vi "clien fix fix.vi"() -> ()   [LabVIEW 2017]
uses:
  <vilib>/Analysis/Matrix/Datatypes/RealMatrix.ctl
  <vilib>/Platform/TimedLoop/XDataNode/timing_clust.ctl
  <vilib>/Platform/TimedLoop/XDataNode/nitl_modes.ctl
  <vilib>/Platform/TimedLoop/XDataNode/wakeup.ctl
  <vilib>/Analysis/Matrix/Numeric/Multiply/Multiply - RM,RM.vi
  <vilib>/platform/TimedLoop/XDataNode/XDataNode.xnode
  <vilib>/Analysis/Matrix/NI_Matrix.lvlib
  <vilib>/Platform/TimedLoop/XDataNode/XDNodeRunTimeDep.lvlib
panel:
  out "appended array":T1
  in  "Array 8":dbl[](array[numeric])
  in  "Array 7":dbl[](array[numeric])
  in  "Array 6":dbl[](array[numeric])
  in  "Array 5":dbl[](array[numeric])
  in  "Array 4":dbl[](array[numeric])
  in  "Array 3":dbl[](array[numeric])
  in  "Array 2":dbl[](array[numeric])
  in  "Array":dbl[](array[numeric])
  in  "Processor 2":i32=-2
  out "Processor":i32=-2
  out "Global End Time":i64
  out "Iteration Duration":i64
  out "?":string="CLIENT"
  out "RESULT":T1
  out "MATRIX FROM SERVER":T1
  in  "Real Matrix":T1
  out "DATA FROM SERVER":i32
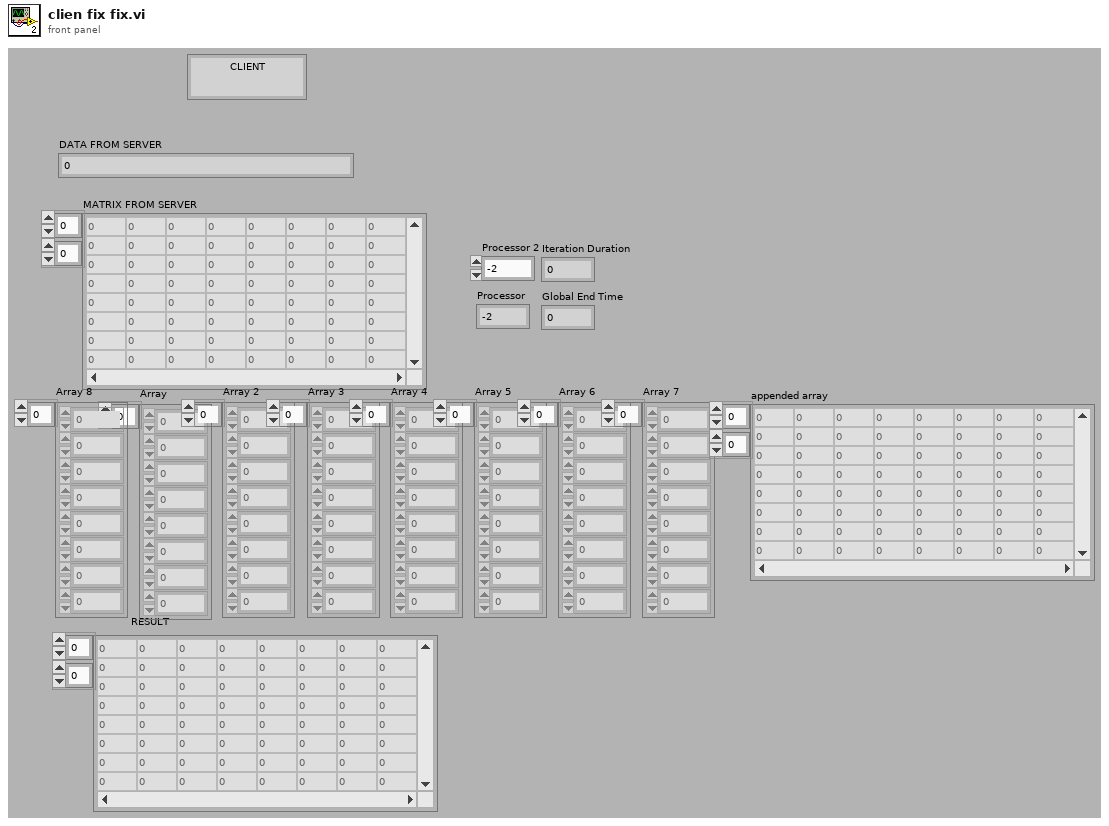
[diagram p1: front panel]
types:
  T1 = typedef "NI_Matrix.lvlib/RealMatrix.ctl" = dbl[][]
  T2 = typedef "XDNodeRunTimeDep.lvlib/timing_clust.ctl" = cluster{"Expected End [f-1]":u64, "Actual End [f-1]":u64, "Finished Late? [f-1]":bool, "Expected End [i-1]":u64, "Actual End [i-1]":u64, "Finished Late? [i-1]":bool, "Expected Start [i]":u64, "Actual Start [i]":u64, "Expected Start [f]":u64, "Actual Start [f]":u64, "Source Name":string, "Structure Name":string, "Period":i64, "Deadline":i64, "Offset":i64, "Start":i64, "Priority":i32, "Timeout":i32, "Mode":T3, "Wakeup Reason":T4, "Error":errorcluster, "Source Type":string, "Secondary Source Type":string, "Global End Time":u64, "Global Start Time":u64, "Frame Duration":u64, "Iteration Duration":u64, "Assigned CPU":i32, "I/O Scan Engine Mode":u32}
  T3 = typedef "XDNodeRunTimeDep.lvlib/nitl_modes.ctl" = enum32{"No Change", "Process missed periods, maintain original phase", "Discard missed periods, maintain original phase", "Process missed periods, ignore original phase", "Discard missed periods, ignore original phase"}
  T4 = typedef "XDNodeRunTimeDep.lvlib/wakeup.ctl" = enum32{"Normal", "Aborted", "Asynchronous wakeup", "Timing source error", "Timed loop error", "Timeout"}
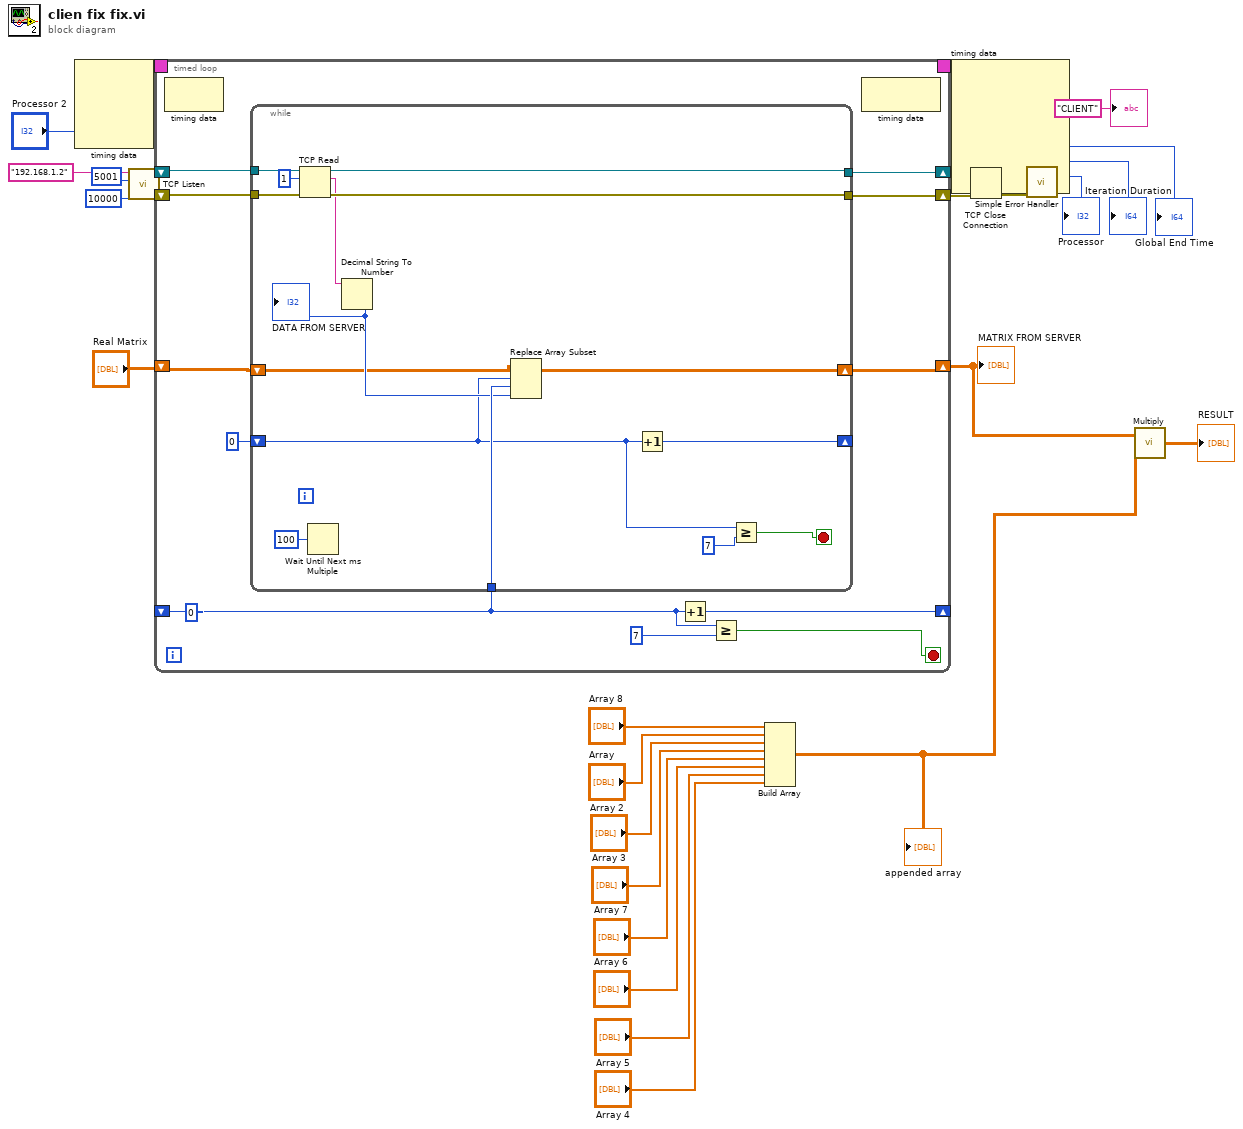
[diagram p0: block diagram]
diagram:
  n1 = node-c288("Processor 2") -> (w16:T2)  [unwired: 3 in]
  n2 = call <vilib>:"TCP Listen.vi"("timeout ms (wait forever: -1)"=10000, "port"=u16 5001, "service name"="192.168.1.2") -> ("error out"=w27:errorcluster, "connection ID"=w28:refnum<k5>)  [unwired: 4 in, 3 out]
  n3 = timed-loop {
    shift-right: [w37] -> w21
    shift-left: w28 -> [w39]
    shift-right: [w36] -> w26
    shift-left: w27 -> [w38]
    shift-right: [w35] -> _
    shift-left: u32 0 ("millisecond multiple") -> [w33]
    shift-right: [w29] -> w19
    shift-left: "Real Matrix" -> [w30]
    timing: w16 -> [_]
    timing-out: [_] -> w15
    stop <- w31 stop-if-true
    n4 = node-c288() -> ()  [unwired: 1 in, 1 out]
    n5 = while {
      tunnel: w39 -> [w56]
      tunnel: w38 -> [w55]
      tunnel: [w53] -> w37
      tunnel: [w51] -> w36
      tunnel: w33 -> [w49]
      shift-right: [w48] -> _
      shift-left: u32 0 ("millisecond multiple") -> [w45]
      shift-right: [w42] -> w29
      shift-left: w30 -> [w43]
      stop <- w46 stop-if-true
      n6 = TCP Read(connection ID=w56, bytes to read=1, error in (no error)=w55) -> (connection ID out=w53:refnum<k5>, data out=w50:string, error out=w51:errorcluster)  [unwired: 2 in]
      n7 = Wait Until Next ms Multiple(millisecond multiple=u32 100) -> ()  [unwired: 1 out]
      n8 = Decimal String To Number(string=w50) -> (number=w47:i32)  [unwired: 2 in, 1 out]
      "DATA FROM SERVER" <- w47
      n9 = Replace Array Subset(array=w43, new element=w47, index (row)=w45, index (col)=w49) -> (w42:T1)
      n10 = Increment(x=w45) -> (x+1=w48:u32)
      n11 = Greater Or Equal?(x=w45, y=u32 7 ("millisecond multiple")) -> (x >= y?=w46:bool)
    }
    n12 = Increment(x=w33) -> (x+1=w35:u32)
    n13 = Greater Or Equal?(x=w33, y=u32 7 ("millisecond multiple")) -> (x >= y?=w31:bool)
    n14 = node-c288() -> ()  [unwired: 1 in, 1 out]
  }
  "MATRIX FROM SERVER" <- w19
  n15 = Build Array("Array 8", "Array", "Array 2", "Array 3", "Array 7", "Array 6", "Array 5", "Array 4") -> (w1:T1)
  "appended array" <- w1
  n16 = node-c288(w15) -> (→"Global End Time":i64, →"Iteration Duration":i64, →"Processor":i32)  [unwired: 4 out]
  n17 = TCP Close Connection(connection ID=w21, error in (no error)=w26) -> (error out=w20:errorcluster)  [unwired: 1 in, 1 out]
  n18 = call <vilib>:"Simple Error Handler.vi"("error in (no error)"=w20) -> ()  [unwired: 4 in, 5 out]
  n19 = call-poly <vilib>:"Multiply.vi"("Real Matrix B"=w1, "Real Matrix A"=w19) -> ("A * B"=→"RESULT":T1)
  "?" <- "CLIENT"
